vi "MCL Print Device Info.vi"(8 "error in (no error)":errorcluster, 11 "handle":i32) -> (0 "error out":errorcluster)   [LabVIEW 2014, in "Madlib.lvlib"]
doc: "MADLIB_API void MCL_PrintDeviceInfo(int handle);"
uses:
  <userlib>/Lambda2/lib/Madlib/Madlib.lvlib
  <userlib>/Lambda2/lib/Madlib/Madlib.dll
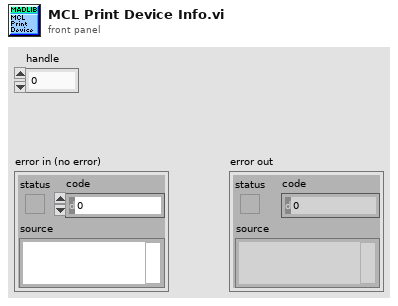
[diagram p1: front panel]
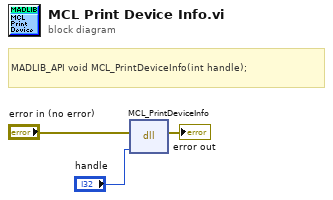
[diagram p0: block diagram]
diagram:
  # "MADLIB_API\tvoid\tMCL_PrintDeviceInfo(int handle);"
  n1 = dll-call lib="C:/Program Files (x86)/National Instruments/LabVIEW 2014/user.lib/Lambda2/lib/Madlib/Madlib.*" fn="MCL_PrintDeviceInfo"(error in="error in (no error)", "handle"="handle") -> (error out=→"error out":errorcluster)  [unwired: 4 in, 1 out]
